vi "Set Channel Group Decimation.vi"(8 "error in":errorcluster, 10 "decimation":i32=1 min=1, 11 "channel group in":T1 format="%.0x") -> (0 "error out":errorcluster, 3 "channel group out":T1 format="%.0x")   [LabVIEW 2027, in "Embedded Data Logger Scripting.lvlib"]
uses:
  Embedded Data Logger Scripting.lvlib
  <vilib>/NI VeriStand/Custom Device API/Custom Device Item Ref.ctl
  Shared/Constants.vi
  <vilib>/NI VeriStand/Custom Device Tools/Custom Device Utility Library/NI VeriStand - Search for Item by GUID.vi
  <vilib>/NI VeriStand/Custom Device Tools/Custom Device Utility Library/Custom Device Utility Library.lvlib
  <vilib>/NI VeriStand/Custom Device API/Custom Device API.lvlib
  Shared/Embedded Data Logger Shared.lvlib
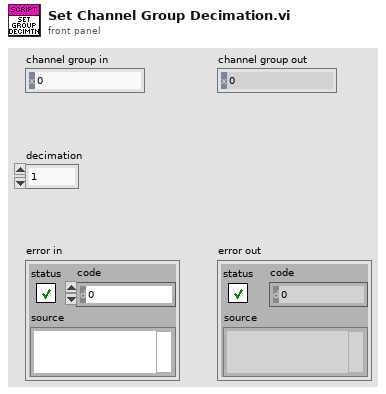
[diagram p1: front panel]
types:
  T1 = typedef "Custom Device API.lvlib/Custom Device Item Ref.ctl" = u64
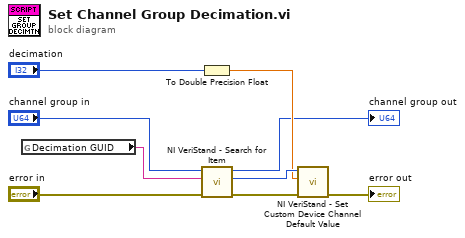
[diagram p0: block diagram]
diagram:
  n1 = global read "Constants.vi" "Decimation GUID"() -> (w7:string)
  n2 = To Double Precision Float(number="decimation") -> (double precision float=w2:dbl)
  n3 = call-poly <vilib>:"NI VeriStand - Search for Item.vi"("error in"="error in", "Item GUID"=w7, "Section Ref in"="channel group in") -> ("error out"=w9:errorcluster, "Item Ref"=w8:T1, "Section Ref out"=→"channel group out":T1)  [unwired: 6 out]
  n4 = call <vilib>:"NI VeriStand - Set Custom Device Channel Default Value.vi"("error in (no error)"=w9, "Default Value"=w2, "Channel Ref in"=w8) -> ("error out"=→"error out":errorcluster)  [unwired: 8 out]
